vi "DBL to FXP Raw.vi"(7 "FXP Configuration":T1, 8 "error in (no error)":errorcluster, 10 "DBL Value":dbl) -> (0 "error out":errorcluster, 2 "Bool Data":bool[](array[boolean]))   [LabVIEW 2020, in "FPGA Register IO.lvlib"]
uses:
  FPGA Register IO.lvlib
  TypeDefs/FXP Configuration.ctl
  <vilib>/fxp/LVFixedPointRepBitsTypeDef.ctl
  <vilib>/fxp/LVFixedPointRepRangeTypeDef.ctl
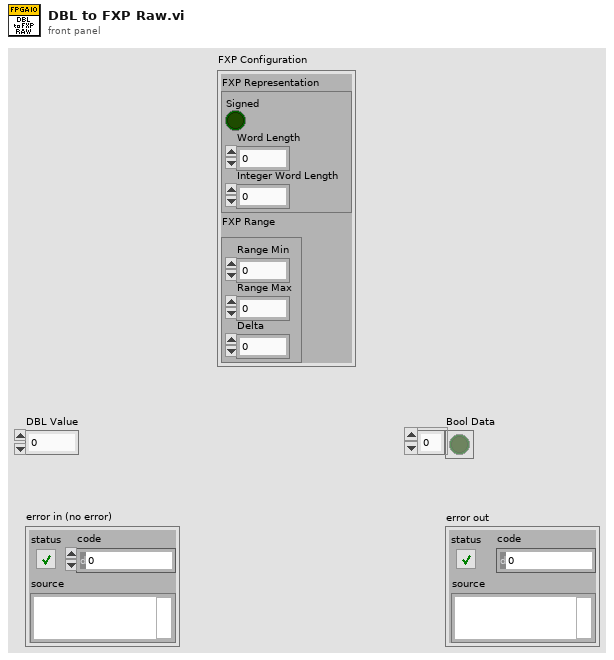
[diagram p1: front panel]
types:
  T1 = typedef "FPGA Register IO.lvlib/FXP Configuration.ctl" = cluster{"FXP Representation":T2, "FXP Range":T3}
  T2 = typedef "LVFixedPointRepBitsTypeDef.ctl" = cluster{"Signed":bool, "Word Length":u32, "Integer Word Length":i32}
  T3 = typedef "LVFixedPointRepRangeTypeDef.ctl" = cluster{"Range Min":dbl, "Range Max":dbl, "Delta":dbl}
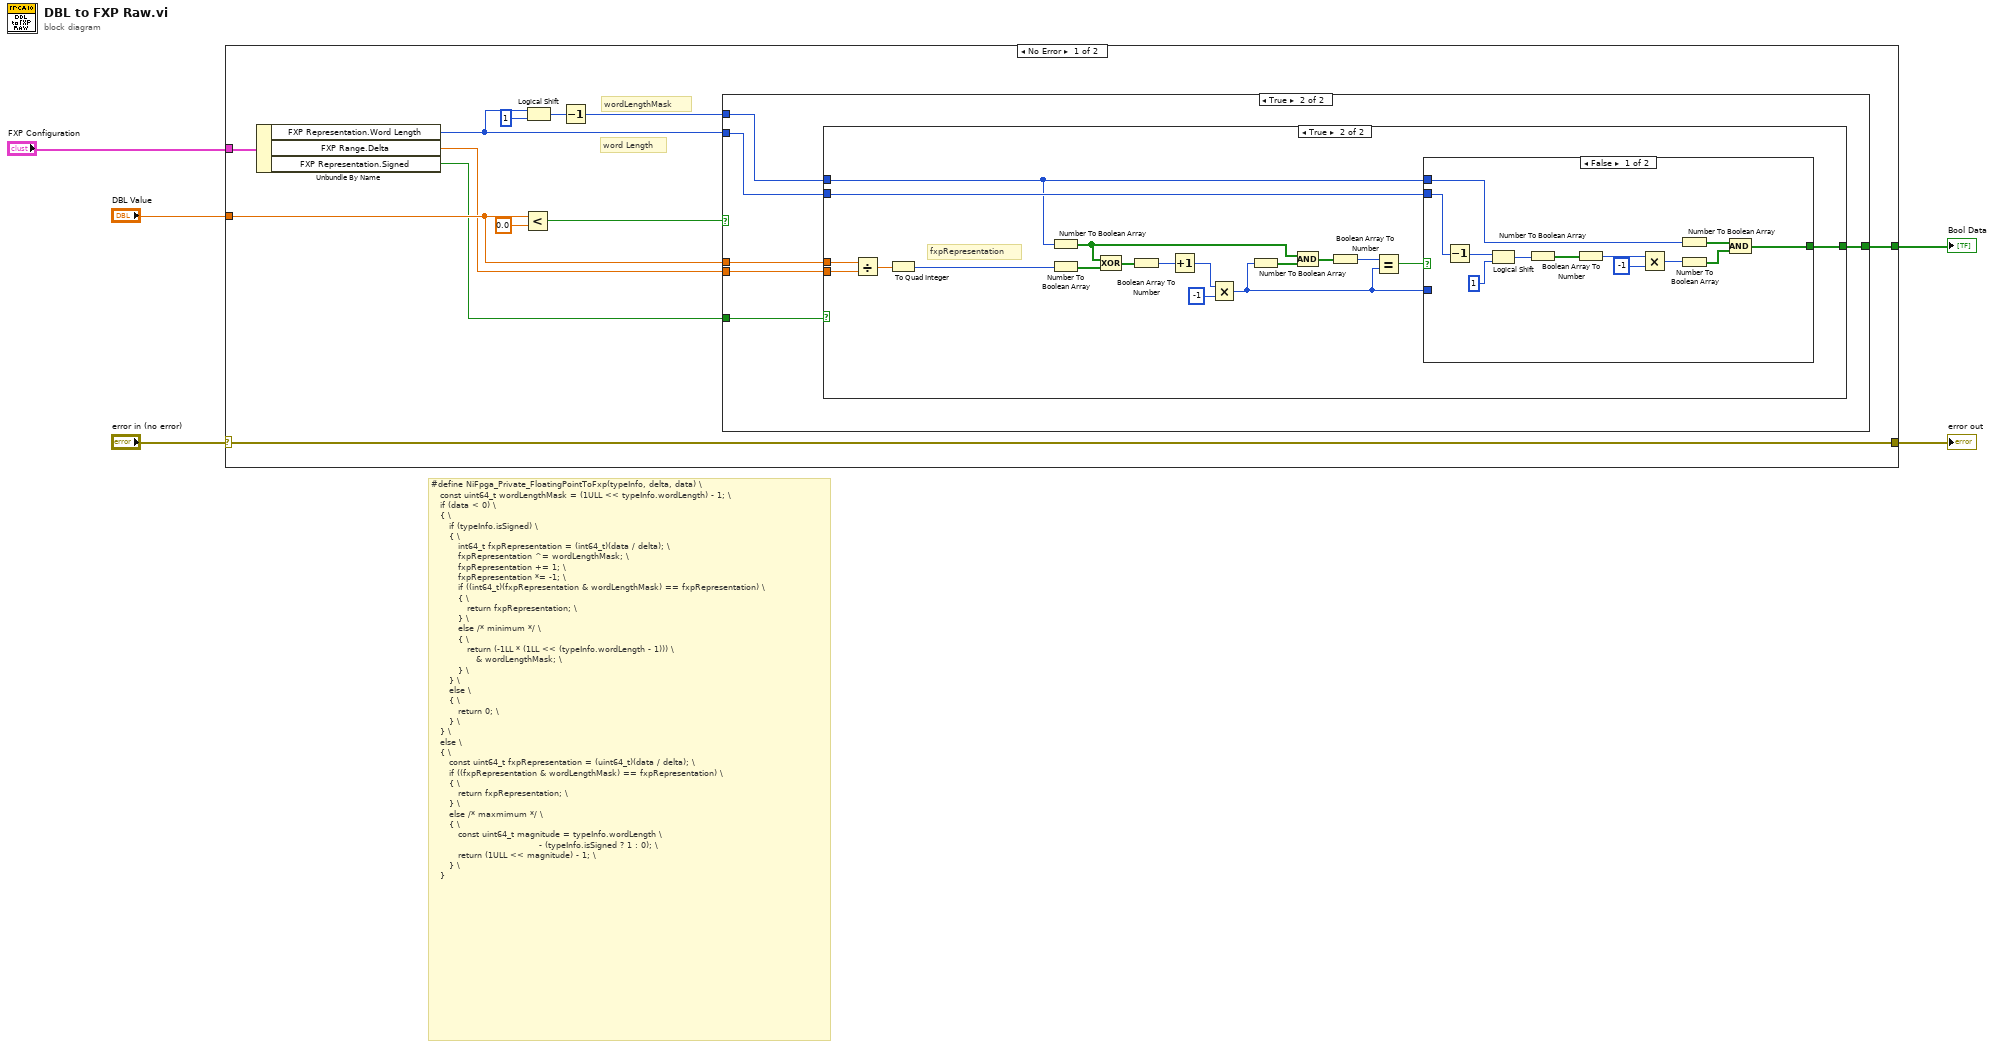
[diagram p0: block diagram]
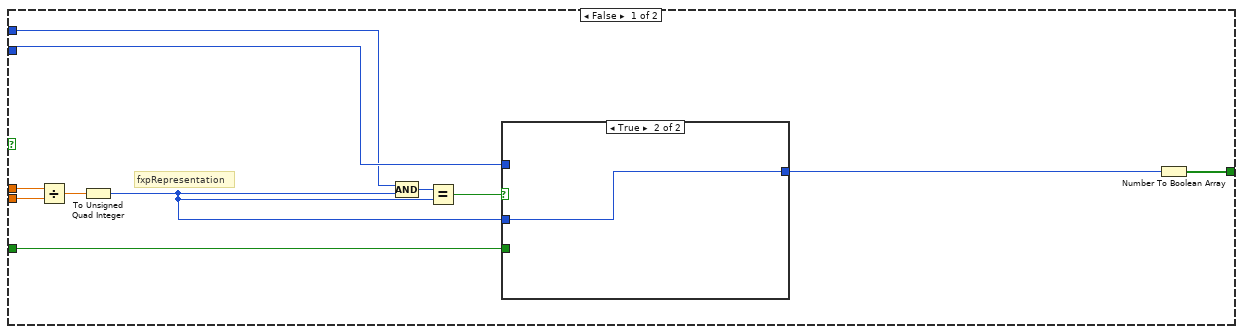
[diagram p2: hidden frame]
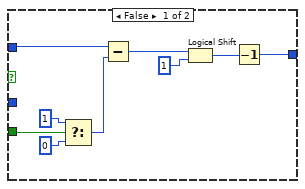
[diagram p3: hidden frame]
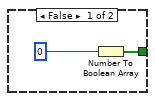
[diagram p4: hidden frame]
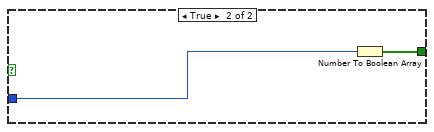
[diagram p5: hidden frame]
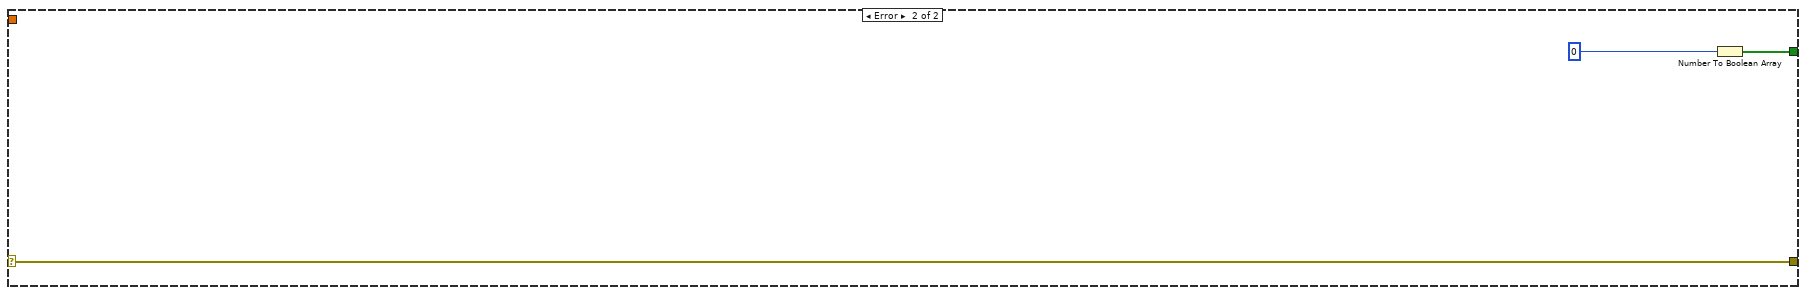
[diagram p6: hidden frame]
diagram:
  # "#define NiFpga_Private_FloatingPointToFxp(typeInfo, delta, data) \\\n   const uint64_t wordLengthMask = (1ULL << typeInfo.wordLength) - 1; \\\n   if (data < 0) \\\n   { \\\n      if (typeInfo.isSigned) \\\n      { \\\n         int64_t fxpRepresentation = (int64_t)(data / delta); \\\n         fxpRepresentation ^= wordLengthMask; \\\n         fxpRepresentation += 1; \\\n         fxpRepresentation *= -1; \\\n         if ((int64_t)(fxpRepresentation & wordLengthMask) == fxpRepresentation) \\\n         { \\\n            return fxpRepresentation; \\\n         } \\\n         else /* minimum */ \\\n         { \\\n            return (-1LL * (1LL << (typeInfo.wordLength - 1))) \\\n               & wordLengthMask; \\\n         } \\\n      } \\\n      else \\\n      { \\\n         return 0; \\\n      } \\\n   } \\\n   else \\\n   { \\\n      const uint64_t fxpRepresentation = (uint64_t)(data / delta); \\\n      if ((fxpRepresentation & wordLengthMask) == fxpRepresentation) \\\n      { \\\n         return fxpRepresentation; \\\n      } \\\n      else /* maxmimum */ \\\n      { \\\n         const uint64_t magnitude = typeInfo.wordLength \\\n                                    - (typeInfo.isSigned ? 1 : 0); \\\n         return (1ULL << magnitude) - 1; \\\n      } \\\n   }"
  n1 = case shown="No Error" "error in (no error)" {
    selector: "error in (no error)" -> [w8 w81]
    tunnel: "FXP Configuration" -> [w12 _]
    tunnel: [w8 w81] -> w4
    tunnel: "DBL Value" -> [w11 _]
    tunnel: [w7 w80] -> w1
    frame No Error {
      # "word Length"
      # "wordLengthMask"
      n2 = Unbundle By Name(w12) -> ("FXP Representation.Word Length"=w6:u32, "FXP Range.Delta"=w10:dbl, "FXP Representation.Signed"=w9:bool)
      n3 = Less?(x=w11, y=0.0) -> (x < y?=w14:bool)
      n4 = Logical Shift(y=w6, x=u64 1) -> (x << y=w17:u64)
      n5 = Decrement(x=w17) -> (x-1=w13:u64)
      n6 = case shown="True" w14 {
        tunnel: w9 -> [w22 w44]
        tunnel: w11 -> [w28 w43]
        tunnel: w10 -> [w27 w42]
        tunnel: w6 -> [w23 w41]
        tunnel: w13 -> [w21 w40]
        tunnel: [w18 w39] -> w7
        frame False {
          # "fxpRepresentation"
          n7 = Divide(x=w28, y=w27) -> (x/y=w26:dbl)
          n8 = To Unsigned Quad Integer(1:w26) -> (0:w20:u64)
          n9 = Compound Arithmetic op=AND(w21, w20) -> (w25:u64)
          n10 = Equal?(x=w25, y=w20) -> (x = y?=w24:bool)
          n11 = case shown="True" w24 {
            tunnel: [w29 w38] -> w19
            tunnel: w23 -> [w34 _]
            tunnel: w22 -> [w37 _]
            tunnel: w20 -> [_ w38]
            frame False {
              n12 = Select(t=u32 1 ("word length"), s=w37, f=u32 0) -> (s? t:f=w33:u32)
              n13 = Subtract(x=w34, y=w33) -> (x-y=w32:u32)
              n14 = Logical Shift(y=w32, x=u64 1) -> (x << y=w30:u64)
              n15 = Decrement(x=w30) -> (x-1=w29:u64)
            }
            frame True {
            }
          }
          n16 = Number To Boolean Array(number=w19) -> (Boolean array=w18:bool[])
        }
        frame True {
          n17 = case shown="True" w44 {
            tunnel: w43 -> [_ w64]
            tunnel: w42 -> [_ w63]
            tunnel: w40 -> [_ w48]
            tunnel: w41 -> [_ w52]
            tunnel: [w46 w47] -> w39
            frame False {
              n18 = Number To Boolean Array(number=i64 0) -> (Boolean array=w46:bool[])
            }
            frame True {
              # "fxpRepresentation"
              n19 = Divide(x=w64, y=w63) -> (x/y=w62:dbl)
              n20 = To Quad Integer(1:w62) -> (0:w61:i64)
              n21 = Number To Boolean Array(number=w48) -> (Boolean array=w56:bool[])
              n22 = Number To Boolean Array(number=w61) -> (Boolean array=w60:bool[])
              n23 = Compound Arithmetic op=XOR(w56, w60) -> (w59:bool[])
              n24 = Boolean Array To Number(Boolean array=w59) -> (number=w58:i64)
              n25 = Increment(x=w58) -> (x+1=w51:i64)
              n26 = Multiply(x=w51, y=i64 -1) -> (x*y=w49:i64)
              n27 = Number To Boolean Array(number=w49) -> (Boolean array=w55:bool[])
              n28 = Compound Arithmetic op=AND(w56, w55) -> (w54:bool[])
              n29 = Boolean Array To Number(Boolean array=w54) -> (number=w50:i64)
              n30 = Equal?(x=w50, y=w49) -> (x = y?=w53:bool)
              n31 = case shown="False" w53 {
                tunnel: w52 -> [w74 _]
                tunnel: w48 -> [w68 _]
                tunnel: w49 -> [_ w78]
                tunnel: [w65 w77] -> w47
                frame False {
                  n32 = Decrement(x=w74) -> (x-1=w75:u32)
                  n33 = Logical Shift(y=w75, x=u64 1) -> (x << y=w73:u64)
                  n34 = Number To Boolean Array(number=w73) -> (Boolean array=w72:bool[])
                  n35 = Boolean Array To Number(Boolean array=w72) -> (number=w71:i64)
                  n36 = Multiply(x=w71, y=i64 -1) -> (x*y=w69:i64)
                  n37 = Number To Boolean Array(number=w68) -> (Boolean array=w67:bool[])
                  n38 = Number To Boolean Array(number=w69) -> (Boolean array=w66:bool[])
                  n39 = Compound Arithmetic op=AND(w67, w66) -> (w65:bool[])
                }
                frame True {
                  n40 = Number To Boolean Array(number=w78) -> (Boolean array=w77:bool[])
                }
              }
            }
          }
        }
      }
    }
    frame Error {
      n41 = Number To Boolean Array(number=u64 0) -> (Boolean array=w80:bool[])
    }
  }
  "error out" <- w4
  "Bool Data" <- w1
